vi "2. vision影像矩陣.vi"() -> ()   [LabVIEW 2014]
uses:
  <vilib>/vision/driver/NI_Vision_Acquisition_Software.lvlib
  <vilib>/vision/NI_Vision_Development_Module.lvlib
panel:
  out "單色影像":T1(plugin-control)
  out "Image Pixels (U8)":u8[][](array[numeric])
  in  "選擇要的顏色":i32(ring)=1 items=["Red", "Green", "Blue", "Hue", "Saturation", "Luminance", "Value", "Intensity"]
  out "彩色影像":T1(plugin-control)
  in  "stop":bool
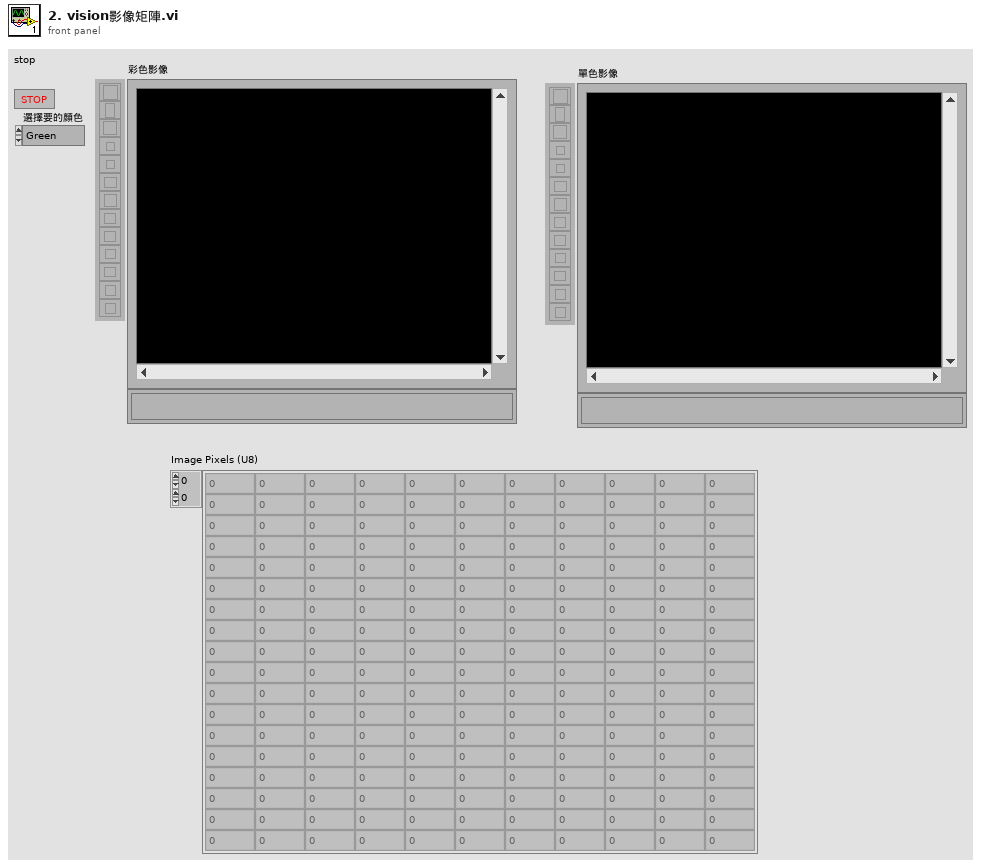
[diagram p1: front panel]
types:
  T1 = typedef "IMAQ Image.ctl" = refnum<image>
  T2 = typedef "Image Type" = u32
  T3 = cluster{"Type":u32, "Version":u32, "Flags":u32, "SerialNumberHigh":u32, "SerialNumberLow":u32, "BusType":u32, "InterfaceName":string, "VendorName":string, "ModelName":string, "CameraFileName":string, "CameraAttributeURL":string}[]
  T4 = cluster{"Type":u32, "Version":u32, "Flags":u32, "SerialNumberHigh":u32, "SerialNumberLow":u32, "BusType":u32, "InterfaceName":string, "VendorName":string, "ModelName":string, "CameraFileName":string, "CameraAttributeURL":string}
  T5 = typedef "IMAQdx.ctl" = refnum<k21>
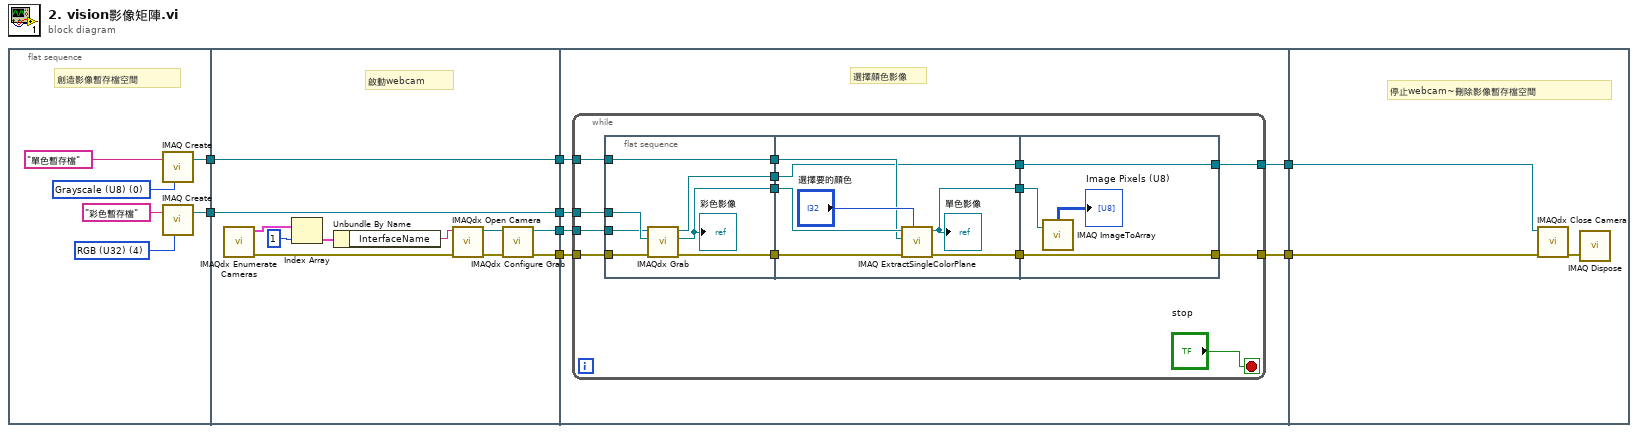
[diagram p0: block diagram]
diagram:
  n1 = flat-sequence {
    tunnel: [w14] -> w8
    tunnel: [w9] -> w7
    tunnel: w8 -> [w25]
    tunnel: w7 -> [w24]
    tunnel: [w25] -> w6
    tunnel: [w24] -> w5
    tunnel: [w16] -> w4
    tunnel: [w15] -> w3
    tunnel: w6 -> [w30]
    tunnel: w5 -> [w31]
    tunnel: w4 -> [w29]
    tunnel: w3 -> [w28]
    tunnel: [w27] -> w2
    tunnel: [w26] -> w1
    tunnel: w2 -> [w64]
    tunnel: w1 -> [w65]
    frame #0 {
      w11 = T2 0 items=["Grayscale (U8)", "Grayscale (I16)", "Grayscale (SGL)", "Complex (CSG)", "RGB (U32)", "HSL (U32)", "RGB (U64)", "Grayscale (U16)"] ("Image Type")
      w13 = T2 4 items=["Grayscale (U8)", "Grayscale (I16)", "Grayscale (SGL)", "Complex (CSG)", "RGB (U32)", "HSL (U32)", "RGB (U64)", "Grayscale (U16)"] ("Image Type")
      # "創造影像暫存檔空間"
      n2 = call "IMAQ Create"("Image Name"="單色暫存檔", "Image Type"=w11) -> ("New Image"=w9:T1)  [unwired: 3 in, 1 out]
      n3 = call "IMAQ Create"("Image Name"="彩色暫存檔", "Image Type"=w13) -> ("New Image"=w14:T1)  [unwired: 3 in, 1 out]
    }
    frame #1 {
      # "啟動webcam"
      n4 = call <vilib>:"IMAQdx Enumerate Cameras.vi"() -> ("error out"=w22:errorcluster, "Camera Information Array"=w17:T3)  [unwired: 10 in]
      n5 = Index Array(array=w17, index=1) -> (element=w20:T4)
      n6 = Unbundle By Name(w20) -> ("InterfaceName"=w18:string)
      n7 = call <vilib>:"IMAQdx Open Camera.vi"("error in"=w22, "Session In"=w18) -> ("error out"=w23:errorcluster, "Session Out"=w21:T5)  [unwired: 8 in]
      n8 = call <vilib>:"IMAQdx Configure Grab.vi"("error in"=w23, "Session In"=w21) -> ("error out"=w15:errorcluster, "Session Out"=w16:T5)  [unwired: 8 in]
    }
    frame #2 {
      # "選擇顏色影像"
      n9 = while {
        tunnel: w31 -> [w34]
        tunnel: w30 -> [w42]
        tunnel: w29 -> [w41]
        tunnel: w28 -> [w40]
        tunnel: [w35] -> w27
        tunnel: [w38] -> w26
        stop <- "stop" stop-if-true
        n10 = flat-sequence {
          tunnel: w42 -> [w52]
          tunnel: w41 -> [w51]
          tunnel: w40 -> [w50]
          tunnel: [w49] -> w39
          tunnel: [w48] -> w37
          tunnel: w34 -> [w47]
          tunnel: [w47] -> w33
          tunnel: [w46] -> w32
          tunnel: [w59] -> w44
          tunnel: [w56] -> w43
          tunnel: w39 -> [w58]
          tunnel: w37 -> [w55]
          tunnel: [w53] -> w36
          tunnel: w33 -> [w54]
          tunnel: w32 -> [w53]
          tunnel: [w63] -> w38
          tunnel: w44 -> [w63]
          tunnel: w43 -> [w61]
          tunnel: [w60] -> w35
          tunnel: w36 -> [w60]
          frame #0 {
            n11 = call <vilib>:"IMAQdx Grab.vi"("error in"=w50, "Image In"=w52, "Session In"=w51) -> ("error out"=w49:errorcluster, "Image Out"=w48:T1, "Session Out"=w46:T5)  [unwired: 5 in, 1 out]
            "彩色影像" <- w48
          }
          frame #1 {
            n12 = call "IMAQ ExtractSingleColorPlane"("Color Plane"="選擇要的顏色", "error in (no error)"=w58, "Image Dst"=w54, "Image Src"=w55) -> ("error out"=w59:errorcluster, "Image Dst Out"=w56:T1)  [unwired: 6 in]
            "單色影像" <- w56
          }
          frame #2 {
            n13 = call "IMAQ ImageToArray"("Image"=w61) -> ("Image Pixels (U8)"=→"Image Pixels (U8)":u8[][])  [unwired: 3 in, 4 out]
          }
        }
      }
    }
    frame #3 {
      # "停止webcam~刪除影像暫存檔空間"
      n14 = call <vilib>:"IMAQdx Close Camera.vi"("error in"=w65, "Session In"=w64) -> ("error out"=w66:errorcluster)  [unwired: 9 in]
      n15 = call "IMAQ Dispose"("error in (no error)"=w66) -> ()  [unwired: 5 in, 1 out]
    }
  }
